vi "Bool Array To Grid Map Test.vi"() -> ()   [LabVIEW 2017]
uses:
  Classes/ElectrodeGrid.lvclass
  Classes/ElectrodeGrid.lvclass/ElectrodeGrid.ctl
panel:
  in  "Array":bool[](array[boolean])
  in  "stop":bool
  out "SM Electrode Grid":bool[][](array[boolean])
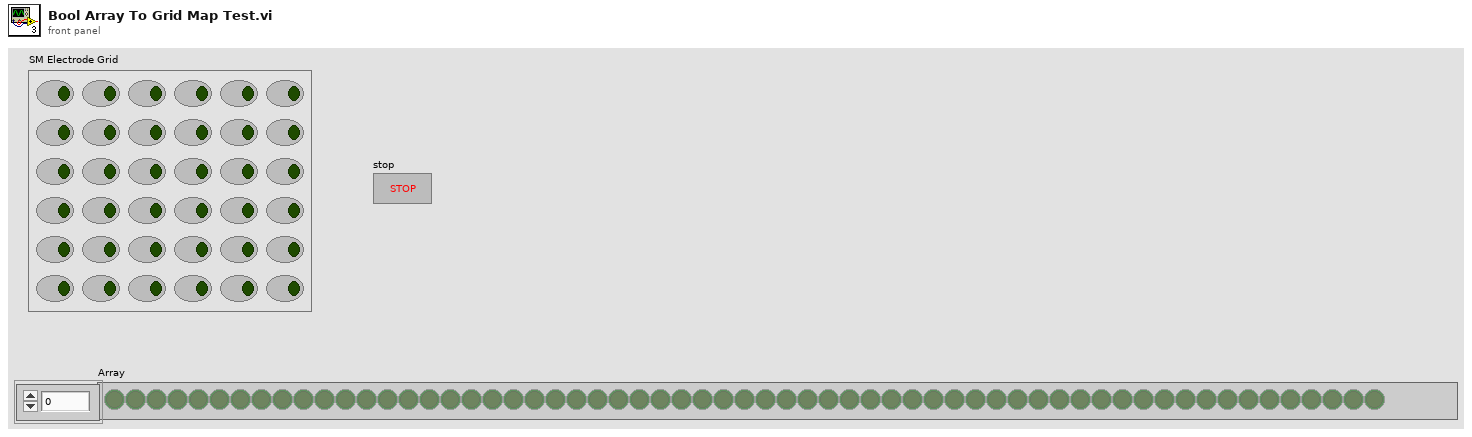
[diagram p1: front panel]
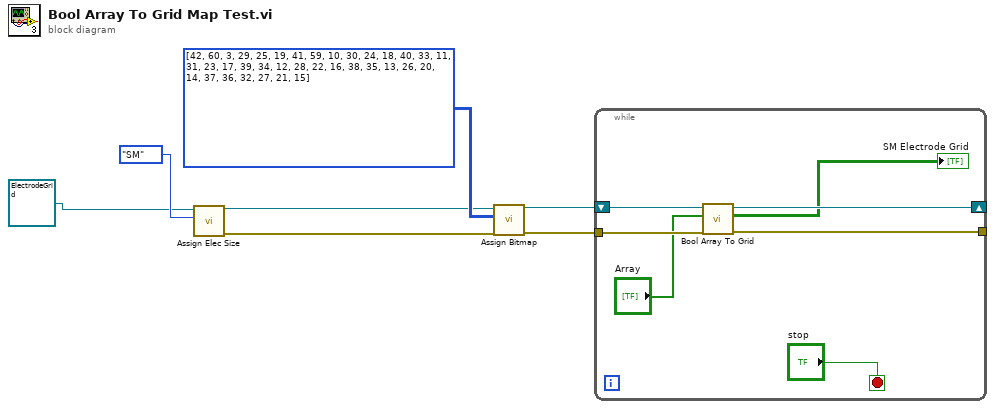
[diagram p0: block diagram]
diagram:
  n1 = call "Assign Elec Size.vi"("electrode size"=enum16{"XS", "SM", "LG"}."SM", "ElectrodeGrid in"=refnum<class "ElectrodeGrid.lvclass"> refnum ("ElectrodeGrid.lvclass")) -> ("error out"=w3:errorcluster, "ElectrodeGrid out"=w2:refnum<class "ElectrodeGrid.lvclass">)  [unwired: 8 in]
  n2 = call "Assign Bitmap.vi"("error in (no error)"=w3, "bitmap"=u8[][] [[42, 60, 3, 29, 25, 19], [41, 59, 10, 30, 24, 18], [40, 33, 11, 31, 23, 17], [39, 34, 12, 28, 22, 16], [38, 35, 13, 26, 20, 14], [37, 36, 32, 27, 21, 15]], "ElectrodeGrid in"=w2) -> ("error out"=w4:errorcluster, "ElectrodeGrid out"=w1:refnum<class "ElectrodeGrid.lvclass">)  [unwired: 7 in]
  n3 = while {
    tunnel: w4 -> [w13]
    shift-right: [w11] -> _
    shift-left: w1 -> [w12]
    tunnel: [w10] -> _
    stop <- "stop" stop-if-true
    n4 = call "Bool Array To Grid.vi"("error in (no error)"=w13, "Bool Array In"="Array", "ElectrodeGrid in"=w12) -> ("error out"=w10:errorcluster, "Elec Grid Output"=→"SM Electrode Grid":bool[][], "ElectrodeGrid out"=w11:refnum<class "ElectrodeGrid.lvclass">)  [unwired: 6 in]
  }
